vi "Shut off Gauge Alarm.vi"(2 "Knob Refnum":refnum<vi>) -> ()   [LabVIEW 2012]
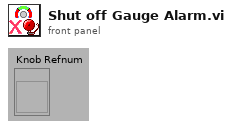
[diagram p1: front panel]
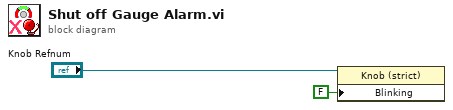
[diagram p0: block diagram]
diagram:
  n1 = property on="Property Node" class="Knob (strict)"(reference="Knob Refnum", "Blinking"=FALSE) -> ()  [unwired: 1 in, 2 out]
